vi "Dereference-String.vi"(8 "No Error":errorcluster, 11 "Str [const char *]":i64 format="%.0x") -> (0 "error out":errorcluster, 3 "String":string)   [LabVIEW 2024, in "SDL3.lvlib" / "LV-Utilities.lvlib"]
doc: "<B>Summary</B>\nDereference <B>Str</B> pointer into <B>String</B>."
uses:
  LV-Utilities.lvlib
  Stdinc/Strlen.vi/60e5867b-eda9-4e5d-b360-fbc458930bd4.vi
  <vilib>/Utility/error.llb/Error Cluster From Error Code.vi
  Stdinc/Stdinc.lvlib
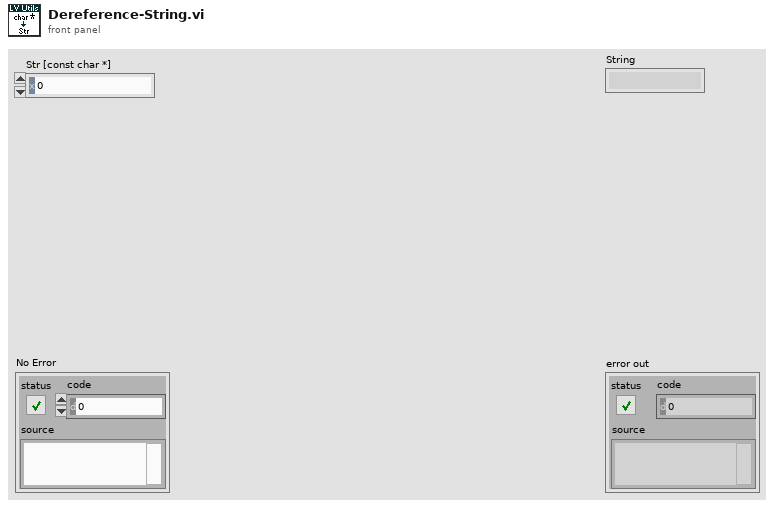
[diagram p1: front panel]
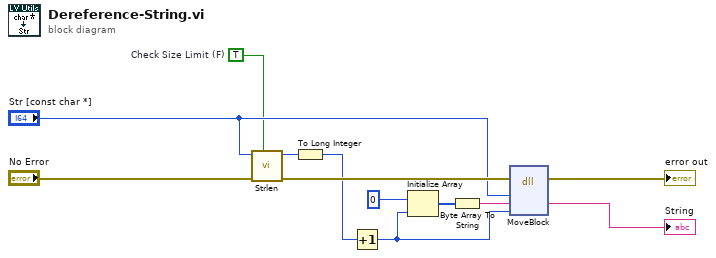
[diagram p0: block diagram]
diagram:
  w3 = TRUE  # Check Size Limit (F)
  n1 = call "Strlen.vi"("Check Size Limit (F)"=w3, "No Error"="No Error", "Str [const char *]"="Str [const char *]") -> ("Error Out"=w12:errorcluster, "Size"=w11:u64)  [unwired: 7 in]
  n2 = To Long Integer(number=w11) -> (32bit integer=w2:i32)
  n3 = Increment(x=w2) -> (x+1=w7:i32)
  n4 = Initialize Array(u8 0, w7) -> (w9:u8[])
  n5 = Byte Array To String(unsigned byte array=w9) -> (string=w8:string)
  n6 = dll-call lib="LabVIEW" fn="MoveBlock"(error in=w12, "Address"="Str [const char *]", "Destination"=w8, "Size"=w7) -> (error out=→"error out":errorcluster, "Destination"=→"String":string)  [unwired: 5 in, 1 out]
